vi "EOL CAN_Send_Single_Message.vi"(4 "Retries":i32=5, 6 "Msg Wait Time":u32=100, 7 "Rx Arbitration Id":u32=402522244 format="%.0x", 8 "Error in":errorcluster, 9 "Tx CAN frame":T1={"timestamp"=timestamp(0 s since 1904-01-01), "payload"=[2, 39, 3, 85, 85, 85, 85, 85], "identifier"=402391172, "type"=0, "extended?"=TRUE, "echo?"=FALSE} {"payload" format="%x"; "timestamp" format="%<%.7X\n%x>T"; "type" items=["CAN Data"=0, "CAN Remote"=1, "CAN Bus Error"=2, "CAN 2.0 Data"=8, "CAN FD Data"=16, "CAN FD+BRS Data"=24, "J1939 Data"=192, "Delay"=224, "Log Trigger"=225, "Start Trigger"=226]; "identifier" format="%x"}, 10 "Read Session in":refnum<k21>, 11 "Write Session in":refnum<k21>) -> (0 "Error out":errorcluster, 1 "Rx Message":u8[](array[numeric]) format="%02x", 2 "spreadsheet string":string, 3 "Response Good?":bool, 5 "TxRx Data":string[][](array[string]))   [LabVIEW 2018]
uses:
  <vilib>/xnet/xnet.llb/XNET Frame CAN.ctl
  <vilib>/xnet/xnet.llb/XNET Frame Type CAN.ctl
  <vilib>/xnet/xnet.llb/XNET Write (Frame CAN).vi
  <vilib>/xnet/xnet.llb/XNET Read (Frame CAN).vi
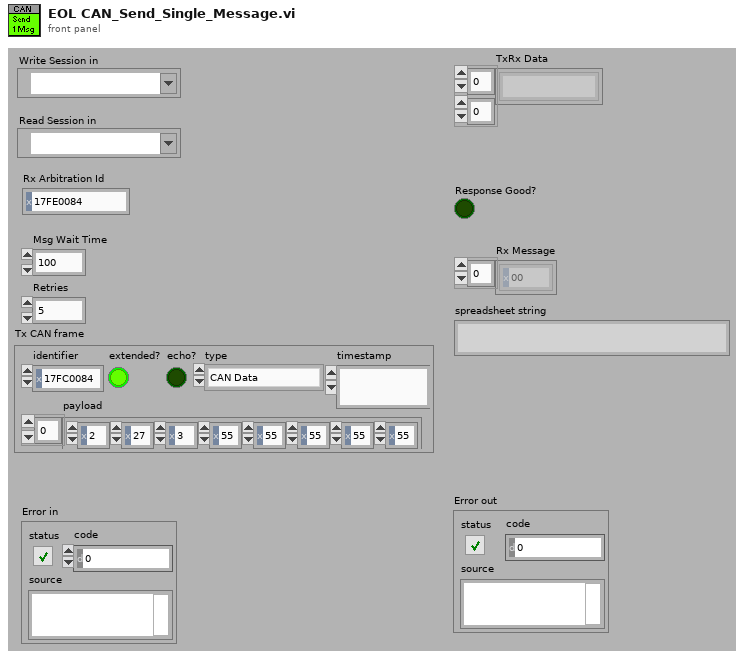
[diagram p1: front panel]
types:
  T1 = typedef "XNET Frame CAN.ctl" = cluster{"timestamp":timestamp, "payload":u8[], "identifier":u32, "type":T2, "extended?":bool, "echo?":bool}
  T2 = typedef "XNET Frame Type CAN.ctl" = u8
  T3 = cluster{"Read Session in":refnum<k21>, "Write Session in":refnum<k21>, "Tx CAN frame":T1, "Rx Arbitration Id":u32, "Retry Counter":i32, "Rx Msg":u8[], "Response Good?":bool, "TxRx Data":string[][], "Message Start Timer":u32, "Message Wait Timer":i32, "Error in":errorcluster}
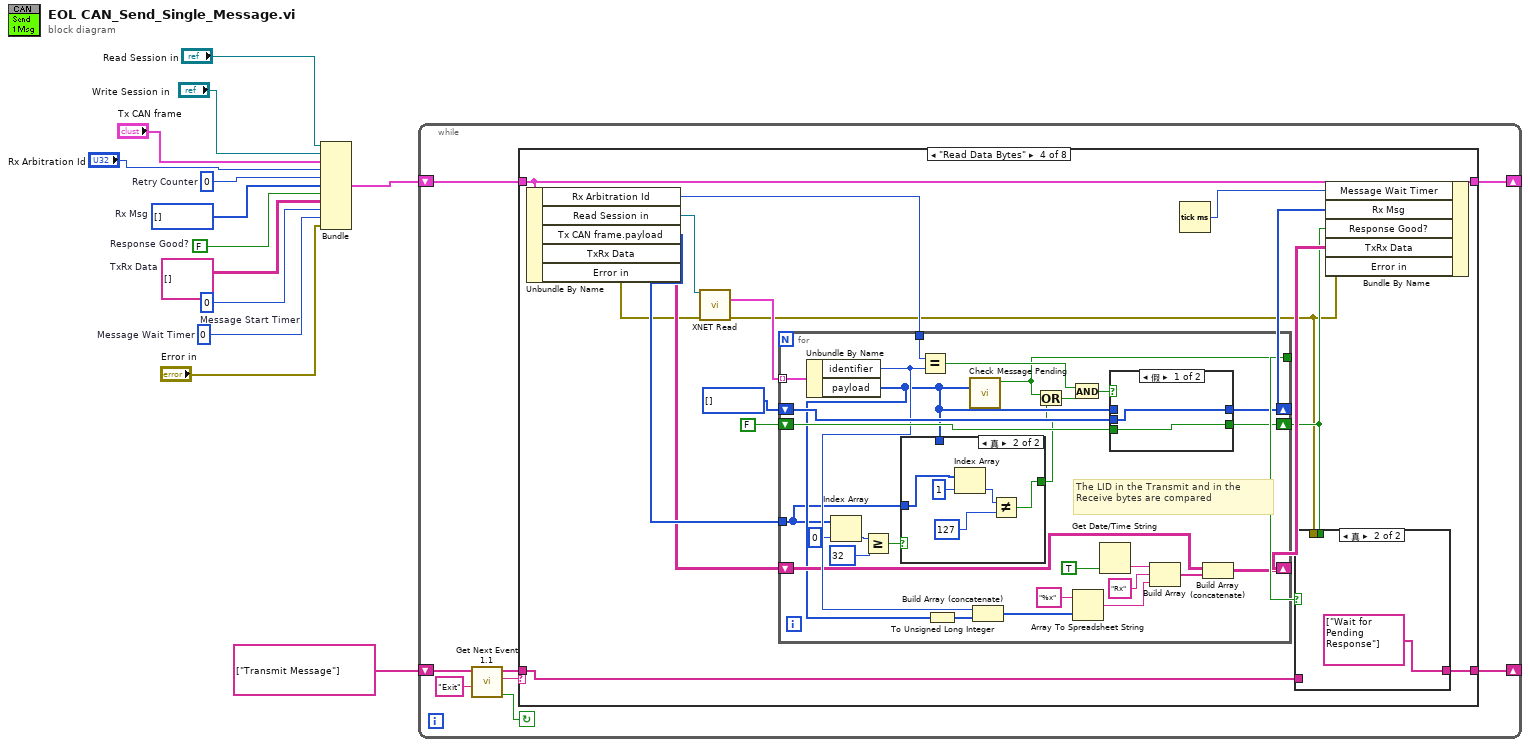
[diagram p0: block diagram]
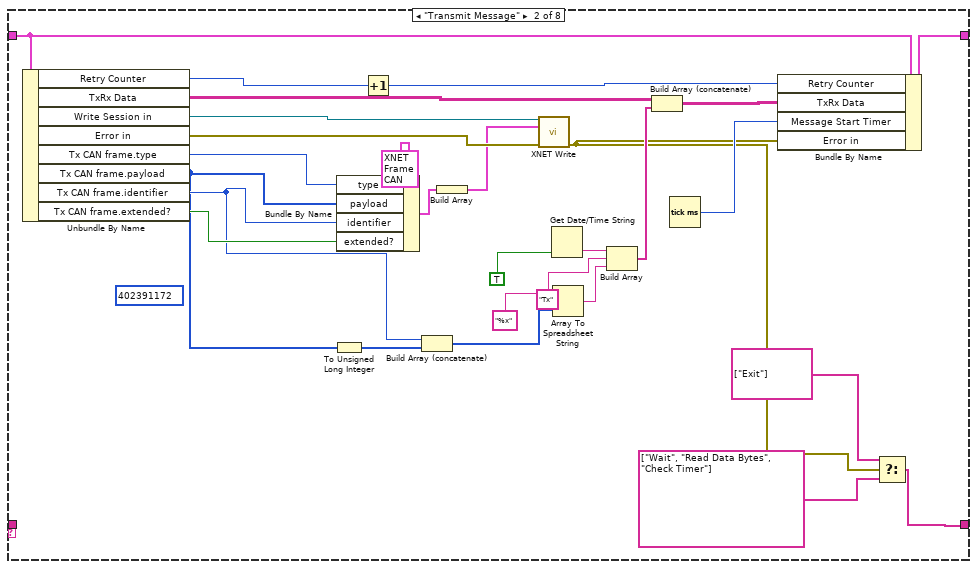
[diagram p3: hidden frame]
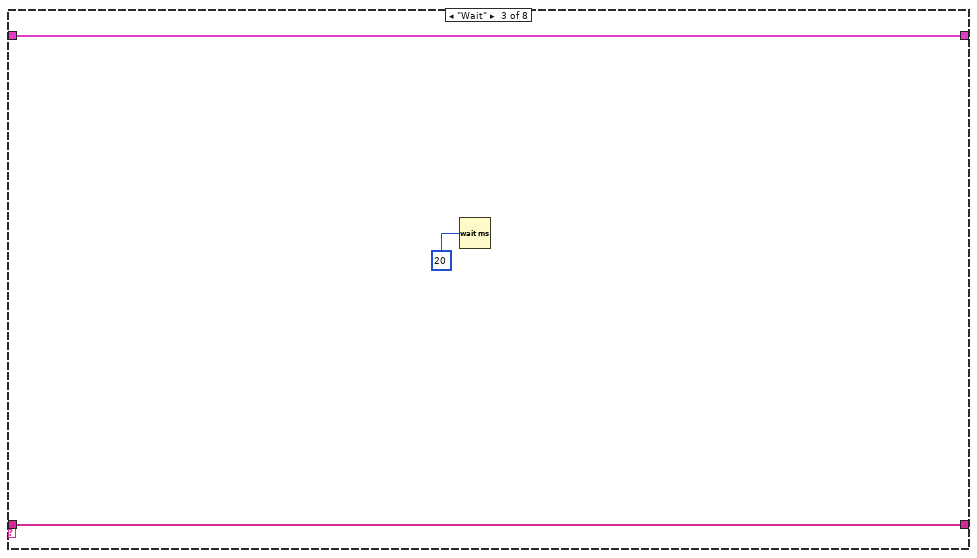
[diagram p4: hidden frame]
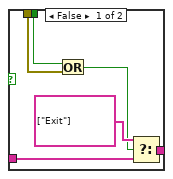
[diagram p5: hidden frame]
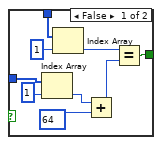
[diagram p6: hidden frame]
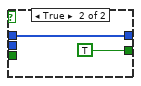
[diagram p7: hidden frame]
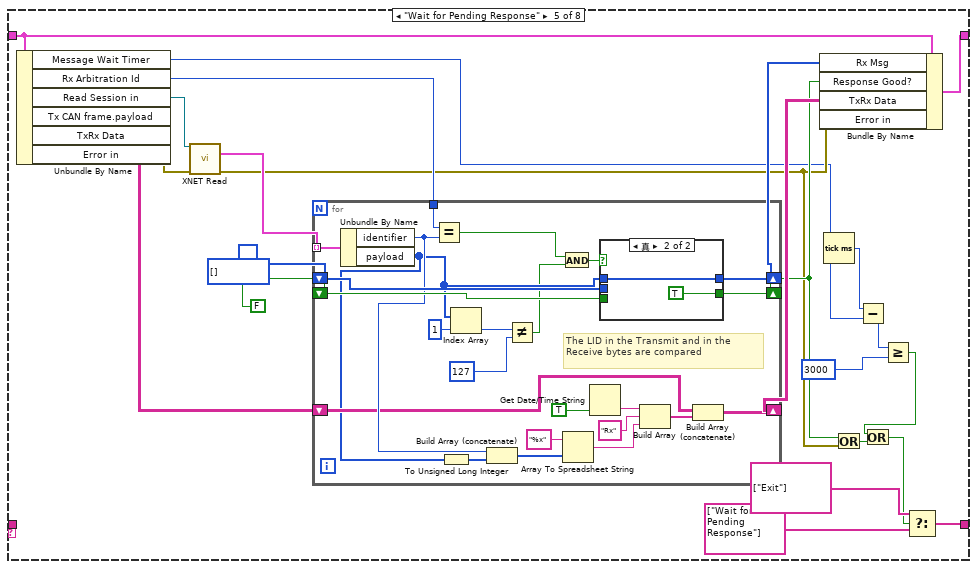
[diagram p8: hidden frame]
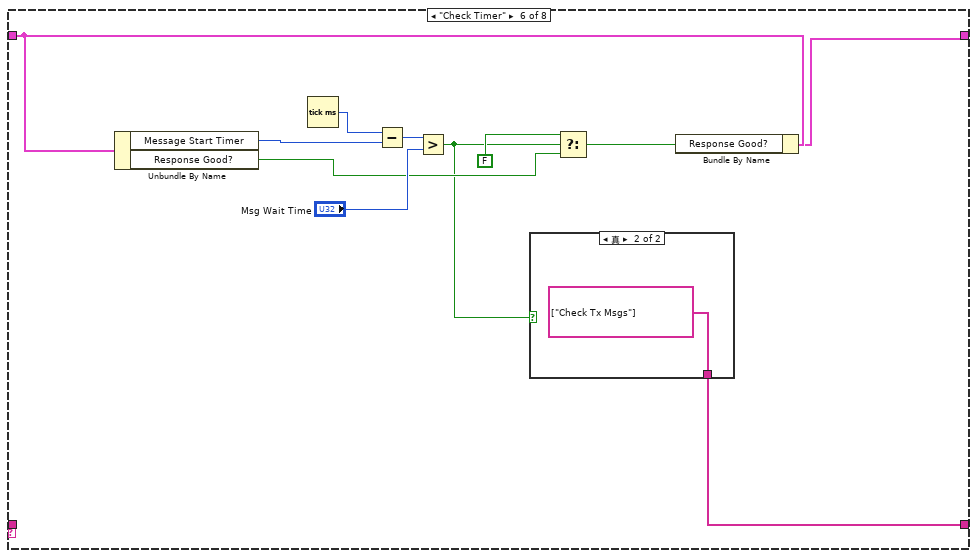
[diagram p10: hidden frame]
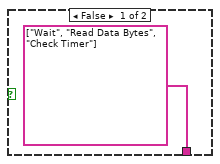
[diagram p11: hidden frame]
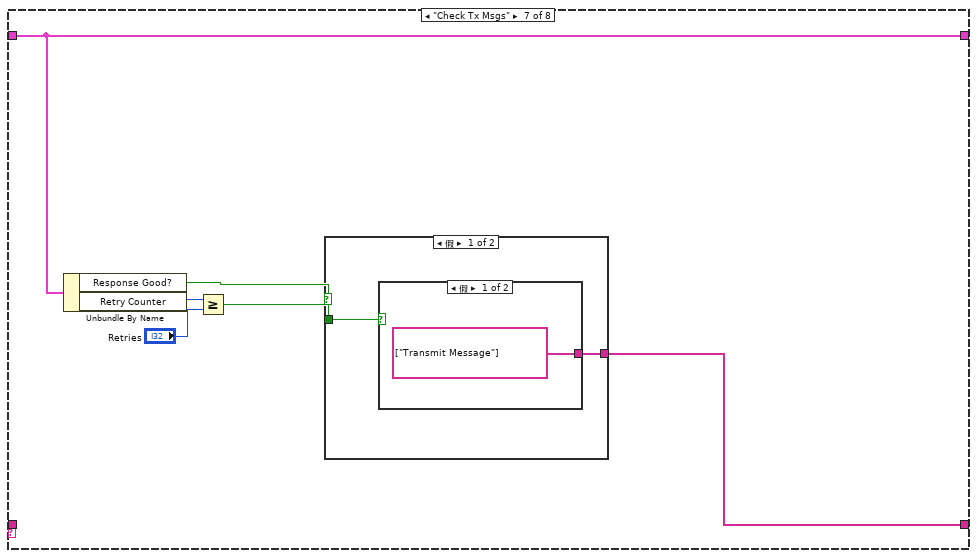
[diagram p12: hidden frame]
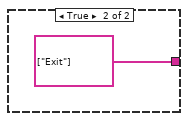
[diagram p13: hidden frame]
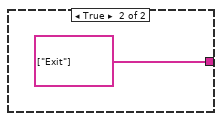
[diagram p14: hidden frame]
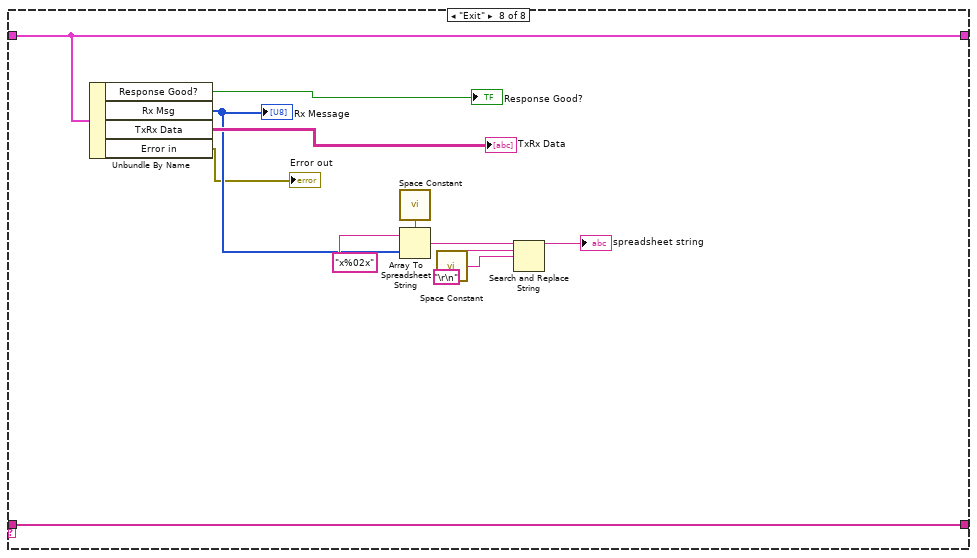
[diagram p15: hidden frame]
diagram:
  w1 = 0  # Message Wait Timer
  w7 = u32 0  # Message Start Timer
  w8 = string[][] []  # TxRx Data
  w9 = FALSE  # Response Good?
  w10 = u8[] []  # Rx Msg
  w12 = 0  # Retry Counter
  n1 = Bundle("Read Session in"="Read Session in", "Write Session in"="Write Session in", "Tx CAN frame"="Tx CAN frame", "Rx Arbitration Id"="Rx Arbitration Id", "Retry Counter"=w12, "Rx Msg"=w10, "Response Good?"=w9, "TxRx Data"=w8, "Message Start Timer"=w7, "Message Wait Timer"=w1, "Error in"="Error in") -> (w11:T3)  [unwired: 1 in]
  n2 = while {
    shift-right: [w18] -> _
    shift-left: string[] ["Transmit Message"] ("event queue out") -> [w17]
    shift-right: [w15] -> _
    shift-left: w11 -> [w16]
    stop <- w21 continue-if-true
    n3 = call "Get Next Event 1.1.vi"("Exit Event"="Exit", "event queue in"=w17) -> ("Condition (Exit:F)"=w21:bool, "next event"=w20:string, "event queue out"=w19:string[])  [unwired: 6 in, 1 out]
    n4 = case shown="\"Transmit Message\"" w20 {
      tunnel: w19 -> [w23 _ w52 w67 _ _ _ w212]
      tunnel: [w23 w27 w52 w66 w144 w177 w192 w212] -> w18
      tunnel: w16 -> [w22 w50 w53 w72 w148 w179 w190 w211]
      tunnel: [w22 w48 w53 w71 w147 w178 w190 w211] -> w15
      frame "Error", Default {
      }
      frame "Transmit Message" {
        (unwired) u32 402391172 ("Tx Arbitration Id")
        n5 = Unbundle By Name(w50) -> ("Retry Counter"=w51:i32, "TxRx Data"=w44:string[][], "Write Session in"=w47:refnum<k21>, "Error in"=w43:errorcluster, "Tx CAN frame.type"=w28:T2, "Tx CAN frame.payload"=w29:u8[], "Tx CAN frame.identifier"=w30:u32, "Tx CAN frame.extended?"=w31:bool)
        n6 = To Unsigned Long Integer(number=w29) -> (unsigned 32bit integer=w42:u32[])
        n7 = Bundle By Name(cluster=T1 {"timestamp"=timestamp(0 s since 1904-01-01), "payload"=[2, 39, 3, 85, 85, 85, 85, 85], "identifier"=402391172, "type"=8, "extended?"=TRUE, "echo?"=FALSE} ("CAN frame"), "type"=w28, "payload"=w29, "identifier"=w30, "extended?"=w31) -> (w34:T1)
        n8 = Increment(x=w51) -> (x+1=w49:i32)
        n9 = Build Array (concatenate)(w30, w42) -> (w36:u32[])
        n10 = Build Array(w34) -> (w32:T1[])
        n11 = call-poly <vilib>:"XNET Write.vi"("session in"=w47, "data"=w32, "error in (no error)"=w43) -> ("error out"=w24:errorcluster)  [unwired: 11 in, 1 out]
        n12 = Get Date/Time String(want seconds? (F)=TRUE) -> (time string=w38:string)  [unwired: 2 in, 1 out]
        n13 = Array To Spreadsheet String(array=w36, 3:"%x" ("format string")) -> (spreadsheet string=w40:string)  [unwired: 1 in]
        n14 = Build Array(w38, "Tx" ("format string"), w40) -> (w41:string[])
        n15 = Build Array (concatenate)(w44, w41) -> (w45:string[][])
        n16 = Tick Count (ms)() -> (millisecond timer value=w46:u32)
        n17 = Bundle By Name(cluster=w50, "Retry Counter"=w49, "TxRx Data"=w45, "Message Start Timer"=w46, "Error in"=w24) -> (w48:T3)
        n18 = Select(t=string[] ["Exit"], s=w24, f=string[] ["Wait", "Read Data Bytes", "Check Timer"] ("event queue out")) -> (s? t:f=w27:string[])
      }
      frame "Wait" {
        n19 = Wait (ms)(milliseconds to wait=u32 20) -> ()  [unwired: 1 out]
      }
      frame "Read Data Bytes" {
        n20 = Unbundle By Name(w72) -> ("Rx Arbitration Id"=w59:u32, "Read Session in"=w69:refnum<k21>, "Tx CAN frame.payload"=w68:u8[], "TxRx Data"=w65:string[][], "Error in"=w63:errorcluster)
        n21 = call-poly <vilib>:"XNET Read.vi"("session in"=w69, "error in (no error)"=w63) -> ("data"=w60:T1[], "error out"=w57:errorcluster)  [unwired: 10 in, 2 out]
        n22 = for {
          tunnel: w60 -> [w107] mode=indexing
          shift-right: [w106] -> w70
          shift-left: u8[] [] ("Data Array") -> [w105]
          shift-right: [w104] -> w58
          shift-left: FALSE -> [w103]
          tunnel: w68 -> [w83]
          shift-right: [w91] -> w64
          shift-left: w65 -> [w92]
          tunnel: w59 -> [w89]
          tunnel: [w85] -> w56
          # "The LID in the Transmit and in the\nReceive bytes are compared"
          n23 = Unbundle By Name(w107) -> ("identifier"=w99:u32, "payload"=w88:u8[])
          n24 = Index Array(array=w83, index=0) -> (element=w82:u8)
          n25 = Greater Or Equal?(x=w82, y=u8 32) -> (x >= y?=w80:bool)
          n26 = case shown="真" w80 {
            tunnel: w88 -> [w113 _]
            tunnel: [w112 w118] -> w87
            tunnel: w83 -> [w111 w117]
            frame False {
              n27 = Index Array(array=w111, index=1) -> (element=w110:u8)
              n28 = Index Array(array=w113, index=1) -> (element=w116:u8)
              n29 = Add(x=w110, y=u8 64 ("Numeric")) -> (x+y=w115:u8)
              n30 = Equal?(x=w116, y=w115) -> (x = y?=w112:bool)
            }
            frame True {
              n31 = Index Array(array=w117, index=1) -> (element=w119:u8)
              n32 = Not Equal?(x=w119, y=u8 127 ("Numeric")) -> (x != y?=w118:bool)
            }
          }
          n33 = Equal?(x=w89, y=w99) -> (x = y?=w101:bool)
          n34 = To Unsigned Long Integer(number=w88) -> (unsigned 32bit integer=w100:u32[])
          n35 = call "Check Message Pending.vi"("Data Array"=w88) -> ("x .and. y?"=w85:bool)  [unwired: 10 in]
          n36 = Build Array (concatenate)(w99, w100) -> (w90:u32[])
          n37 = Or(x=w85, y=w87) -> (x .or. y?=w86:bool)
          n38 = And(x=w101, y=w86) -> (x .and. y?=w102:bool)
          n39 = Array To Spreadsheet String(array=w90, 3:"%x" ("format string")) -> (spreadsheet string=w94:string)  [unwired: 1 in]
          n40 = Get Date/Time String(want seconds? (F)=TRUE) -> (time string=w96:string)  [unwired: 2 in, 1 out]
          n41 = case shown="假" w102 {
            tunnel: w88 -> [_ w124]
            tunnel: [w122 w124] -> w106
            tunnel: w105 -> [w122 _]
            tunnel: [w123 TRUE] -> w104
            tunnel: w103 -> [w123 _]
            frame False {
            }
            frame True {
            }
          }
          n42 = Build Array(w96, "Rx" ("format string"), w94) -> (w93:string[])
          n43 = Build Array (concatenate)(w92, w93) -> (w91:string[][])
        }
        n44 = Tick Count (ms)() -> (millisecond timer value=w55:u32)
        n45 = case shown="真" w56 {
          tunnel: w67 -> [w78 _]
          tunnel: [w77 string[] ["Wait for Pending Response"] ("t")] -> w66
          tunnel: w58 -> [w75 _]
          tunnel: w57 -> [w73 _]
          frame False {
            n46 = Or(x=w75, y=w73) -> (x .or. y?=w74:bool)
            n47 = Select(t=string[] ["Exit"], s=w74, f=w78) -> (s? t:f=w77:string[])
          }
          frame True {
          }
        }
        n48 = Bundle By Name(cluster=w72, "Message Wait Timer"=w55, "Rx Msg"=w70, "Response Good?"=w58, "TxRx Data"=w64, "Error in"=w57) -> (w71:T3)
      }
      frame "Wait for Pending Response" {
        n49 = Unbundle By Name(w148) -> ("Message Wait Timer"=w130:i32, "Rx Arbitration Id"=w137:u32, "Read Session in"=w145:refnum<k21>, "TxRx Data"=w143:string[][], "Error in"=w141:errorcluster)  [unwired: 1 out]
        n50 = call-poly <vilib>:"XNET Read.vi"("session in"=w145, "error in (no error)"=w141) -> ("data"=w138:T1[], "error out"=w135:errorcluster)  [unwired: 10 in, 2 out]
        n51 = for {
          tunnel: w138 -> [w172] mode=indexing
          shift-right: [w171] -> w146
          shift-left: u8[] [] ("Data Array") -> [w170]
          shift-right: [w169] -> w136
          shift-left: FALSE -> [w168]
          shift-right: [w154] -> w142
          shift-left: w143 -> [w155]
          tunnel: w137 -> [w152]
          # "The LID in the Transmit and in the\nReceive bytes are compared"
          n52 = Unbundle By Name(w172) -> ("identifier"=w162:u32, "payload"=w151:u8[])
          n53 = Equal?(x=w152, y=w162) -> (x = y?=w166:bool)
          n54 = To Unsigned Long Integer(number=w151) -> (unsigned 32bit integer=w163:u32[])
          n55 = Index Array(array=w151, index=1) -> (element=w165:u8)
          n56 = Build Array (concatenate)(w162, w163) -> (w153:u32[])
          n57 = Not Equal?(x=w165, y=u8 127 ("Numeric")) -> (x != y?=w150:bool)
          n58 = And(x=w166, y=w150) -> (x .and. y?=w167:bool)
          n59 = Array To Spreadsheet String(array=w153, 3:"%x" ("format string")) -> (spreadsheet string=w157:string)  [unwired: 1 in]
          n60 = Get Date/Time String(want seconds? (F)=TRUE) -> (time string=w159:string)  [unwired: 2 in, 1 out]
          n61 = case shown="真" w167 {
            tunnel: w151 -> [_ w175]
            tunnel: [w174 w175] -> w171
            tunnel: w170 -> [w174 _]
            tunnel: [w173 TRUE] -> w169
            tunnel: w168 -> [w173 _]
            frame False {
            }
            frame True {
            }
          }
          n62 = Build Array(w159, "Rx" ("format string"), w157) -> (w156:string[])
          n63 = Build Array (concatenate)(w155, w156) -> (w154:string[][])
        }
        n64 = Bundle By Name(cluster=w148, "Rx Msg"=w146, "Response Good?"=w136, "TxRx Data"=w142, "Error in"=w135) -> (w147:T3)
        n65 = Tick Count (ms)() -> (millisecond timer value=w129:u32)
        n66 = Or(x=w136, y=w135) -> (x .or. y?=w132:bool)
        n67 = Subtract(x=w129, y=w130) -> (x-y=w128:u32)
        n68 = Greater Or Equal?(x=w128, y=u32 3000) -> (x >= y?=w127:bool)
        n69 = Or(x=w127, y=w132) -> (x .or. y?=w131:bool)
        n70 = Select(t=string[] ["Exit"], s=w131, f=string[] ["Wait for Pending Response"] ("t")) -> (s? t:f=w144:string[])
      }
      frame "Check Timer" {
        n71 = Unbundle By Name(w179) -> ("Message Start Timer"=w186:u32, "Response Good?"=w182:bool)
        n72 = Tick Count (ms)() -> (millisecond timer value=w187:u32)
        n73 = Subtract(x=w187, y=w186) -> (x-y=w185:u32)
        n74 = Greater?(x=w185, y="Msg Wait Time") -> (0:w180:bool)
        n75 = case shown="真" w180 {
          tunnel: [string[] ["Wait", "Read Data Bytes", "Check Timer"] ("event queue out") string[] ["Check Tx Msgs"] ("Events to Insert")] -> w177
          frame False {
          }
          frame True {
          }
        }
        n76 = Select(t=FALSE, s=w180, f=w182) -> (s? t:f=w181:bool)
        n77 = Bundle By Name(cluster=w179, "Response Good?"=w181) -> (w178:T3)
      }
      frame "Check Tx Msgs" {
        n78 = Unbundle By Name(w190) -> ("Response Good?"=w193:bool, "Retry Counter"=w194:i32)
        n79 = Greater Or Equal?(x=w194, y="Retries") -> (x >= y?=w191:bool)
        n80 = case shown="假" w193 {
          tunnel: [w196 string[] ["Exit"] ("event queue out")] -> w192
          tunnel: w191 -> [w197 _]
          frame False {
            n81 = case shown="假" w197 {
              tunnel: [string[] ["Transmit Message"] ("f") string[] ["Exit"] ("event queue out")] -> w196
              frame False {
              }
              frame True {
              }
            }
          }
          frame True {
          }
        }
      }
      frame "Exit" {
        n82 = Unbundle By Name(w211) -> ("Response Good?"=→"Response Good?":bool, "Rx Msg"=w203:u8[], "TxRx Data"=→"TxRx Data":string[][], "Error in"=→"Error out":errorcluster)
        "Rx Message" <- w203
        n83 = call <vilib>:"Space Constant.vi"() -> ("String"=w205:string)
        n84 = Array To Spreadsheet String(delimiter (Tab)=w205, array=w203, 3:"x%02x" ("format string")) -> (spreadsheet string=w204:string)
        n85 = call <vilib>:"Space Constant.vi"() -> ("String"=w207:string)
        n86 = Search and Replace String(input string=w204, search string="\r\n", replace string=w207) -> (result string=→"spreadsheet string":string)  [unwired: 5 in, 3 out]
      }
    }
  }
